vi "get image array subset.vi"(7 "force reset shift registers":bool, 8 "no.of.channels":dbl, 10 "image array in":u16[][][](array[numeric]), 11 "save channels":bool[](array[boolean]) caption="CH 1  CH 2  CH 3  CH 4  CH 5") -> (3 "image array out for save":u16[][][](array[numeric]))   [LabVIEW 2012]
doc: "SciScan 1.2 160622"
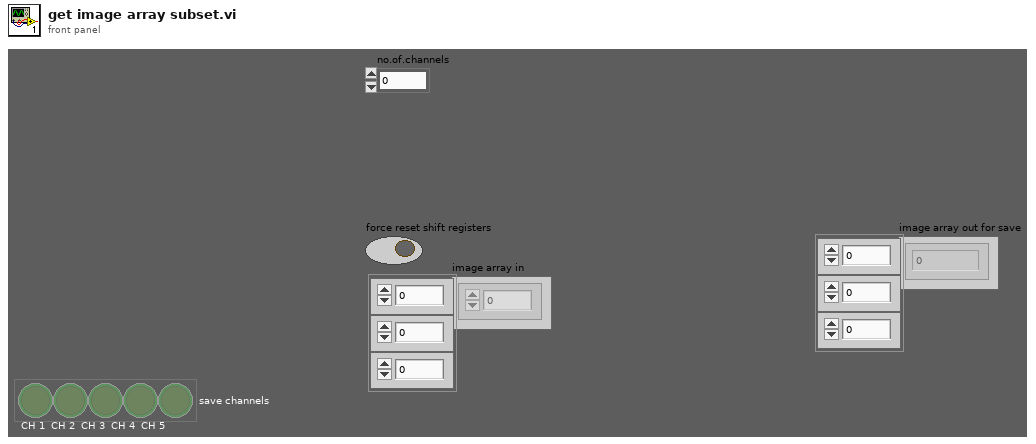
[diagram p1: front panel]
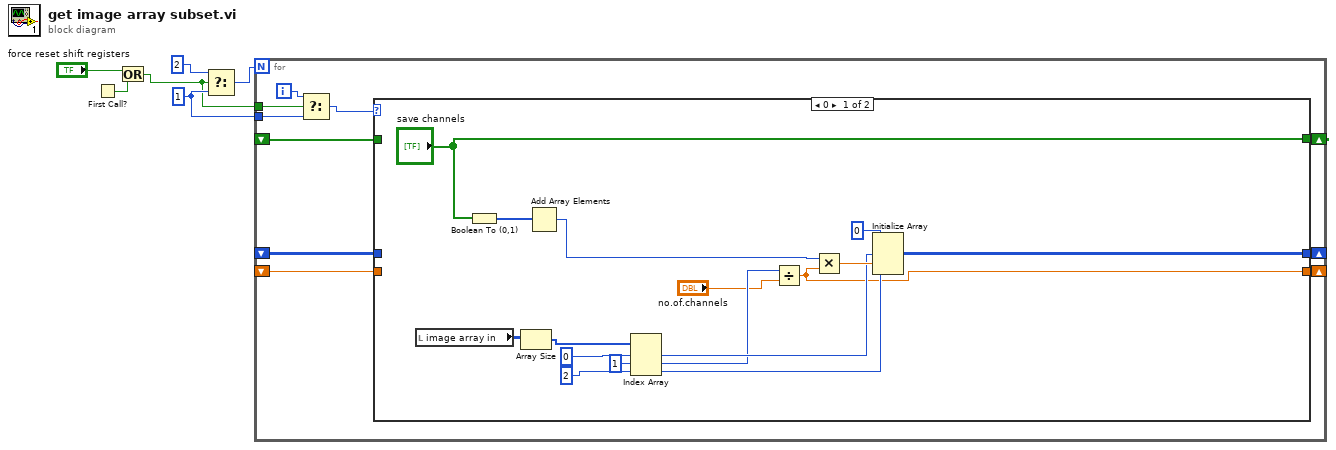
[diagram p0: block diagram]
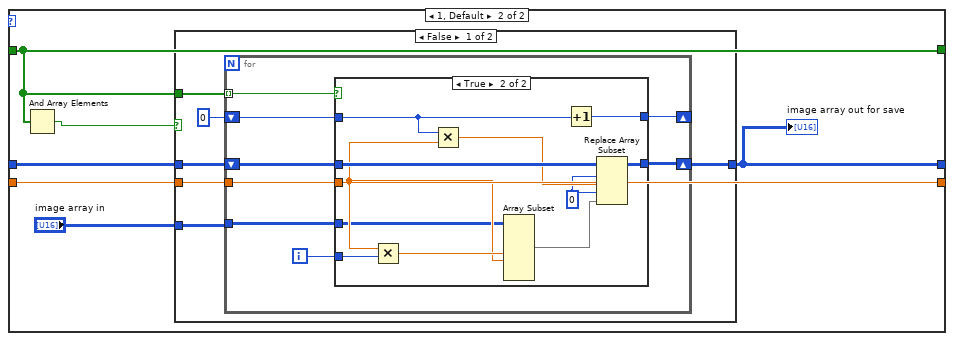
[diagram p2: hidden frame]
diagram:
  w6 = i16 1 ("sum")
  n1 = First Call?() -> (First Call?: T/F=w2:bool)
  n2 = Or(x="force reset shift registers", y=w2) -> (x .or. y?=w5:bool)
  n3 = Select(t=i16 2 ("sum"), s=w5, f=w6) -> (s? t:f=w4:i16)
  n4 = for {
    N: w4 -> [_]
    shift-right: [w14] -> _
    shift-left: _ -> [w15]
    shift-right: [w12] -> _
    shift-left: _ -> [w16]
    shift-right: [w11] -> _
    shift-left: _ -> [w13]
    tunnel: w5 -> [w9]
    tunnel: w6 -> [w8]
    i -> [w10]
    n5 = Select(t=w10, s=w9, f=w8) -> (s? t:f=w7:i32)
    n6 = case shown="0" w7 {
      tunnel: w16 -> [_ w34]
      tunnel: w15 -> [_ w38]
      tunnel: [w31 w35] -> w14
      tunnel: w13 -> [_ w37]
      tunnel: ["save channels" w34] -> w12
      tunnel: [w17 w37] -> w11
      frame 0 {
        n7 = local read "image array in"() -> (w26:u16[][][])
        n8 = Boolean To (0,1)(Boolean="save channels") -> (0, 1=w30:i16[])
        n9 = Array Size(array=w26) -> (size(s)=w25:i32[])
        n10 = Add Array Elements(numeric array=w30) -> (sum=w29:i16)
        n11 = Index Array(array=w25, index #1=0 ("index"), index #2=1 ("index"), index #3=2 ("index")) -> (element #1=w23:i32, element #2=w19:i32, element #3=w21:i32)
        n12 = Divide(x=w19, y="no.of.channels") -> (x/y=w17:dbl)
        n13 = Multiply(x=w29, y=w17) -> (x*y=w28:dbl)
        n14 = Initialize Array(u16 0 ("sum"), w23, w28, w21) -> (w31:u16[][][])
      }
      frame 1, Default {
        n15 = And Array Elements(Boolean array=w34) -> (logical AND=w33:bool)
        n16 = case shown="False" w33 {
          tunnel: w38 -> [w44 _]
          tunnel: w37 -> [w43 _]
          tunnel: "image array in" -> [w42 w66]
          tunnel: [w40 w66] -> w35
          tunnel: w34 -> [w39 _]
          frame False {
            n17 = for {
              tunnel: w39 -> [w52] mode=indexing
              shift-right: [w50] -> w40
              shift-left: w44 -> [w51]
              tunnel: w43 -> [w49]
              tunnel: w42 -> [w48]
              shift-right: [w45] -> _
              shift-left: 0 -> [w46]
              i -> [w47]
              n18 = case shown="True" w52 {
                tunnel: w51 -> [w54 w65]
                tunnel: [w54 w63] -> w50
                tunnel: w49 -> [_ w59]
                tunnel: w48 -> [_ w55]
                tunnel: w47 -> [_ w58]
                tunnel: w46 -> [w53 w62]
                tunnel: [w53 w64] -> w45
                frame False {
                }
                frame True {
                  w57 = 0 ("disabled index (page)")
                  n19 = Multiply(x=w59, y=w58) -> (x*y=w60:dbl)
                  n20 = Multiply(x=w62, y=w59) -> (x*y=w61:dbl)
                  n21 = Array Subset(array=w55, index (dim 1)=w60, length (dim 1)=w59) -> (w56:u16[][][])  [unwired: 4 in]
                  n22 = Increment(x=w62) -> (x+1=w64:i32)
                  n23 = Replace Array Subset(array=w65, new element=w56, index (dim 0)=w57, index (dim 1)=w61, index (dim 2)=w57) -> (w63:u16[][][])
                }
              }
            }
          }
          frame True {
          }
        }
        "image array out for save" <- w35
      }
    }
  }
